vi "Get Keystroke.vi"(11 "Variables and Memory in":T1 {"GFX" format="%02x"}) -> (3 "Variables and Memory out":T1 {"GFX" format="%02x"})   [LabVIEW 2018]
uses:
  Controls/ClusterF.ctl
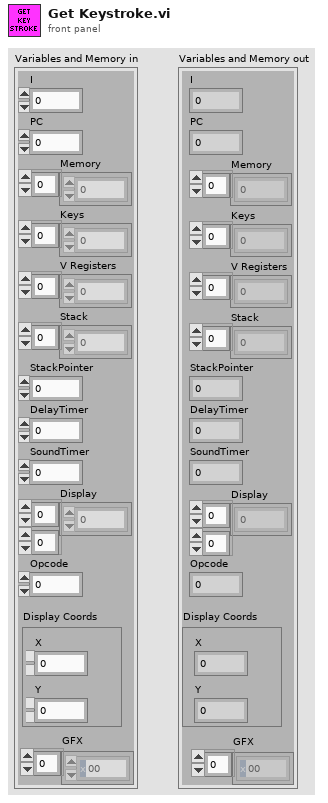
[diagram p1: front panel]
types:
  T1 = typedef "ClusterF.ctl" = cluster{"I":u16, "PC":u16, "Memory":u8[], "Keys":u8[], "V Registers":u8[], "Stack":u16[], "StackPointer":u16, "DelayTimer":u8, "SoundTimer":u8, "Display":u8[][], "Opcode":u16, "Display Coords":cluster{"X":u8, "Y":u8}, "GFX":u8[]}
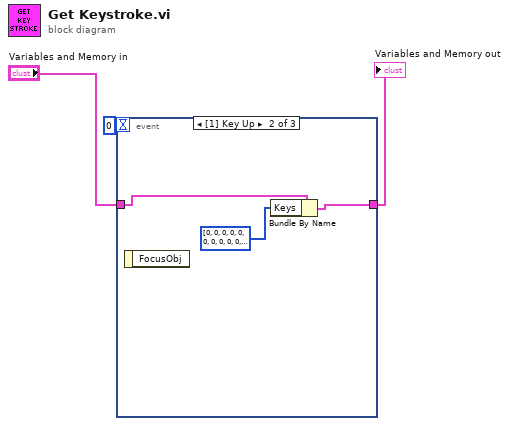
[diagram p0: block diagram]
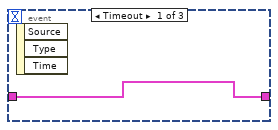
[diagram p2: hidden frame]
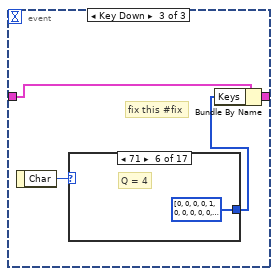
[diagram p3: hidden frame]
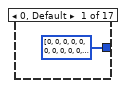
[diagram p4: hidden frame]
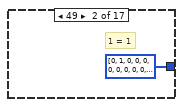
[diagram p5: hidden frame]
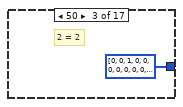
[diagram p6: hidden frame]
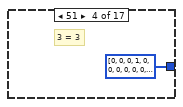
[diagram p7: hidden frame]
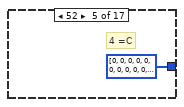
[diagram p8: hidden frame]
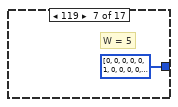
[diagram p9: hidden frame]
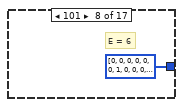
[diagram p10: hidden frame]
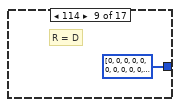
[diagram p11: hidden frame]
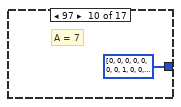
[diagram p12: hidden frame]
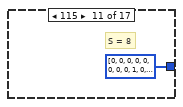
[diagram p13: hidden frame]
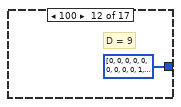
[diagram p14: hidden frame]
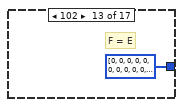
[diagram p15: hidden frame]
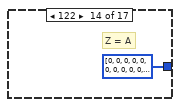
[diagram p16: hidden frame]
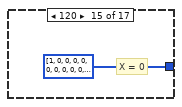
[diagram p17: hidden frame]
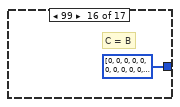
[diagram p18: hidden frame]
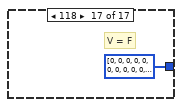
[diagram p19: hidden frame]
diagram:
  n1 = event shown="[1] Key Up" {
    selector: _ -> [_ _ _]
    dyn-events: _ -> [_ _ _]
    timeout: 0 -> [_ _ _]
    tunnel: "Variables and Memory in" -> [w4 w7 w10]
    tunnel: [w4 w5 w11] -> w2
    event Timeout {
      n2 = event-data() -> ()  [unwired: 1 in, 3 out]
    }
    event Key Up {
      n3 = event-data() -> ()  [unwired: 1 in, 1 out]
      n4 = Bundle By Name(cluster=w7, "Keys"=u8[] [0, 0, 0, 0, 0, 0, 0, 0, 0, 0, 0, 0, 0, 0, 0, 0]) -> (w5:T1)
    }
    event Key Down {
      # "fix this #fix"
      n5 = event-data() -> ("Char"=w9:i16)  [unwired: 1 in]
      n6 = case shown="71" w9 {
        tunnel: [u8[] [0, 0, 0, 0, 0, 0, 0, 0, 0, 0, 0, 0, 0, 0, 0, 0] ("Keys 2") u8[] [0, 1, 0, 0, 0, 0, 0, 0, 0, 0, 0, 0, 0, 0, 0, 0] ("Keys 2") u8[] [0, 0, 1, 0, 0, 0, 0, 0, 0, 0, 0, 0, 0, 0, 0, 0] ("Keys 2") u8[] [0, 0, 0, 1, 0, 0, 0, 0, 0, 0, 0, 0, 0, 0, 0, 0] ("Keys 2") u8[] [0, 0, 0, 0, 0, 0, 0, 0, 0, 0, 0, 0, 1, 0, 0, 0] ("Keys 2") u8[] [0, 0, 0, 0, 1, 0, 0, 0, 0, 0, 0, 0, 0, 0, 0, 0] ("Keys 2") u8[] [0, 0, 0, 0, 0, 1, 0, 0, 0, 0, 0, 0, 0, 0, 0, 0] ("Keys 2") u8[] [0, 0, 0, 0, 0, 0, 1, 0, 0, 0, 0, 0, 0, 0, 0, 0] ("Keys 2") u8[] [0, 0, 0, 0, 0, 0, 0, 0, 0, 0, 0, 0, 0, 1, 0, 0] ("Keys 2") u8[] [0, 0, 0, 0, 0, 0, 0, 1, 0, 0, 0, 0, 0, 0, 0, 0] ("Keys 2") u8[] [0, 0, 0, 0, 0, 0, 0, 0, 1, 0, 0, 0, 0, 0, 0, 0] ("Keys 2") u8[] [0, 0, 0, 0, 0, 0, 0, 0, 0, 1, 0, 0, 0, 0, 0, 0] ("Keys 2") u8[] [0, 0, 0, 0, 0, 0, 0, 0, 0, 0, 0, 0, 0, 0, 1, 0] ("Keys 2") u8[] [0, 0, 0, 0, 0, 0, 0, 0, 0, 0, 1, 0, 0, 0, 0, 0] ("Keys 2") u8[] [1, 0, 0, 0, 0, 0, 0, 0, 0, 0, 0, 0, 0, 0, 0, 0] ("Keys 2") u8[] [0, 0, 0, 0, 0, 0, 0, 0, 0, 0, 0, 1, 0, 0, 0, 0] ("Keys 2") u8[] [0, 0, 0, 0, 0, 0, 0, 0, 0, 0, 0, 0, 0, 0, 0, 1] ("Keys 2")] -> w8
        frame 0, Default {
        }
        frame 49 {
          # "1 = 1"
        }
        frame 50 {
          # "2 = 2"
        }
        frame 51 {
          # "3 = 3"
        }
        frame 52 {
          # "4 =C"
        }
        frame 113 {
          # "Q = 4"
        }
        frame 119 {
          # "W = 5"
        }
        frame 101 {
          # "E = 6"
        }
        frame 114 {
          # "R = D"
        }
        frame 97 {
          # "A = 7"
        }
        frame 115 {
          # "S = 8"
        }
        frame 100 {
          # "D = 9"
        }
        frame 102 {
          # "F = E"
        }
        frame 122 {
          # "Z = A"
        }
        frame 120 {
          # "X = 0"
        }
        frame 99 {
          # "C = B"
        }
        frame 118 {
          # "V = F"
        }
      }
      n7 = Bundle By Name(cluster=w10, "Keys"=w8) -> (w11:T1)
    }
  }
  "Variables and Memory out" <- w2
